vi "Write Simulated.vi"(8 "error in (no error)":errorcluster, 10 "Simulated":bool, 11 "Init Parameters in":refnum<class "Init Parameters.lvclass">) -> (0 "error out":errorcluster, 3 "Init Parameters out":refnum<class "Init Parameters.lvclass">)   [LabVIEW 2020, in "%DEVICE% Messaging.lvlib" / "Init Parameters.lvclass"]
uses:
  Init Parameters.lvclass
  Init Parameters.lvclass/Init Parameters.ctl
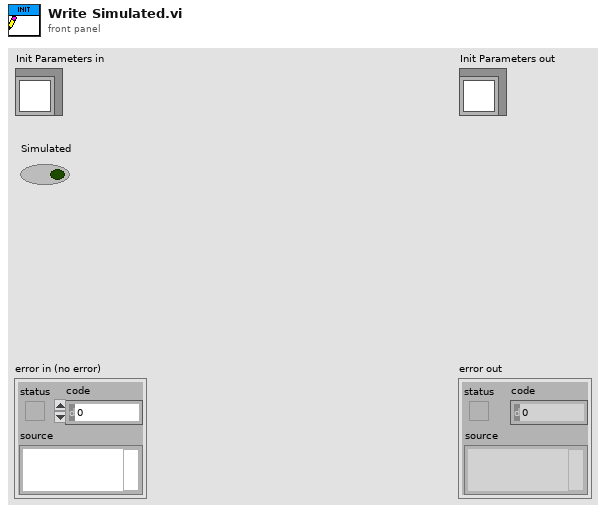
[diagram p1: front panel]
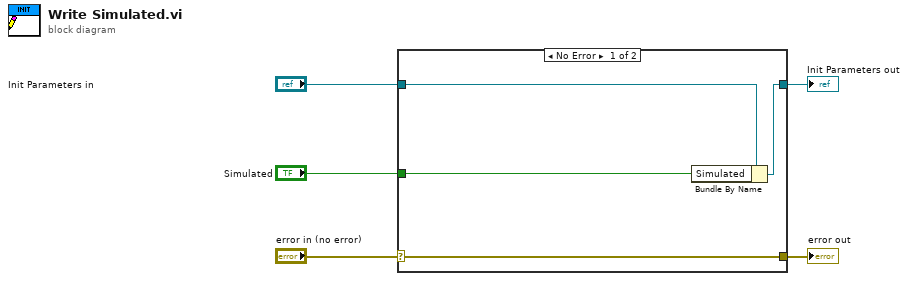
[diagram p0: block diagram]
diagram:
  n1 = case shown="No Error" "error in (no error)" {
    selector: "error in (no error)" -> [w9 w10]
    tunnel: [w9 w10] -> w4
    tunnel: [w7 w11] -> w2
    tunnel: "Init Parameters in" -> [w8 w11]
    tunnel: "Simulated" -> [w6 _]
    frame No Error {
      n2 = Bundle By Name(cluster=w8, "Simulated"=w6) -> (w7:refnum<class "Init Parameters.lvclass">)
    }
    frame Error {
    }
  }
  "error out" <- w4
  "Init Parameters out" <- w2
